vi "Global HEWH.vi"() -> ()   [LabVIEW 2012]
panel:
  in  "Power Labels":string[](array[string])=["VL1", "VL2", "IL1", "IL2", "P", "WH", "Ipeak", "Phi(1,2)"]
  in  "Server IP":string="Unitialized"
  out "MW100 Labels and Chanels":string[][](array[string])
  in  "Midea Data Locations":i32[](array[numeric])=[0, 2, 4, 6, 8, 10, 11, 12, 13, 14, 15, 16]
  in  "Midea Data Fields Logged":string[](array[string])=["Time", "UpperElement", "LowerElement", "Compressor", "Fan1RPM", "Fan2RPM", "SetPoint", "T2(TankSensor)", "T3A(EvapIn)", "T3B(EvapOut)", "T4(CompressorDischarge)", "T5(Ambient)"]
  in  "GEA2 Data Fields":string[](array[string])=["Board Address", "UpperElement", "LowerElement", "Compressor", "Fan", "SetPoint", "T2(TankSensor)", "T3A(EvapIn)", "T3B(EvapOut)", "T4(CompressorDischarge)", "T5(Ambient)", "Current", "Voltage", "EEV", "Hex", "Com Err Count"]
  in  "Test Station:":string="Unitialized"
  in  "Test Number*:":string="T12345678"
  in  "TR Number*:":string="T12345678"
  in  "Unit*:":string="DGnn"
  in  "Comments:":string="R134A Charge Level: 50g"
  in  "Technician:":string="RonR."
  in  "Engineer:":string="CraigT."
  in  "Setup Info:":string="Mode: EHEAT"
  in  "Model*:":string="DGnn"
  in  "Midea Fault Hyperdata":string="0:0:0 UE 24 LE 24 COMP 0 FAN1 0 FAN2 0 SP:0 0 0 0 0 0 C030"
  in  "GEA2 Fault Hyperdata":string="GEA2 256 1 1 2 3 4 5 6 7 8 9 1 2 3 0xee 10"
  out "Tank Flow (GPM,Percent)":dbl[][](array[numeric])
  out "Purge Flow (GPM,Percent)":dbl[][](array[numeric])
  in  "Discarded MW100 Array Data":i32[](array[numeric])=[3, 7, 8, 9, 23, 24, 25, 26, 28, 29, 30, 31, 32, 34]
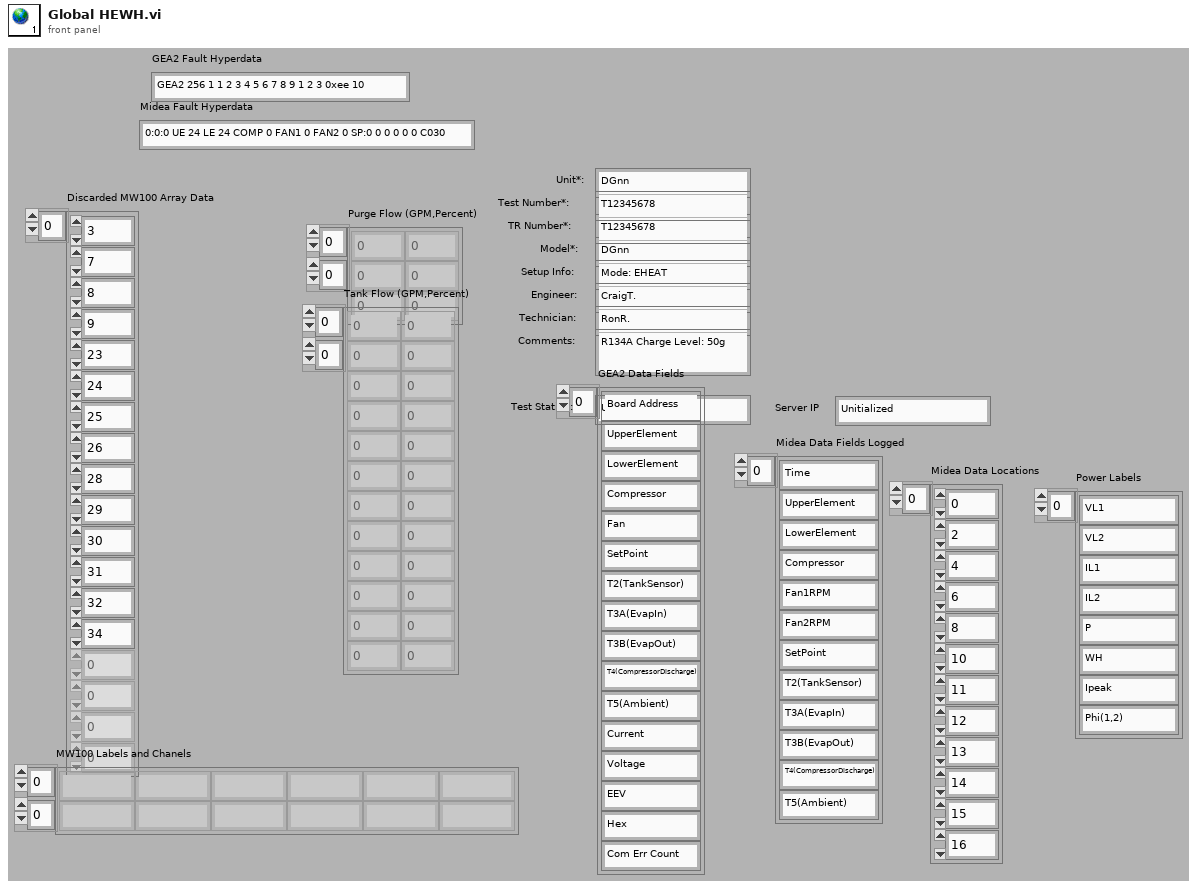
[diagram p1: front panel]
diagram:
